vi "Search_Replace_File.vi"(2 "Replace_String":string="ADC Frequency Hz\t20000", 3 "Search_String":string="ADC Frequency Hz\t1000", 4 "Path":path) -> (0 "error out":errorcluster, 1 "Number Found":i32)   [LabVIEW 2010]
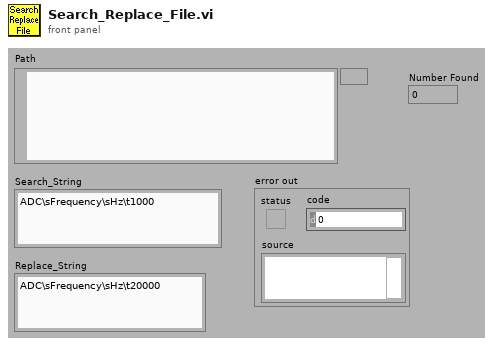
[diagram p1: front panel]
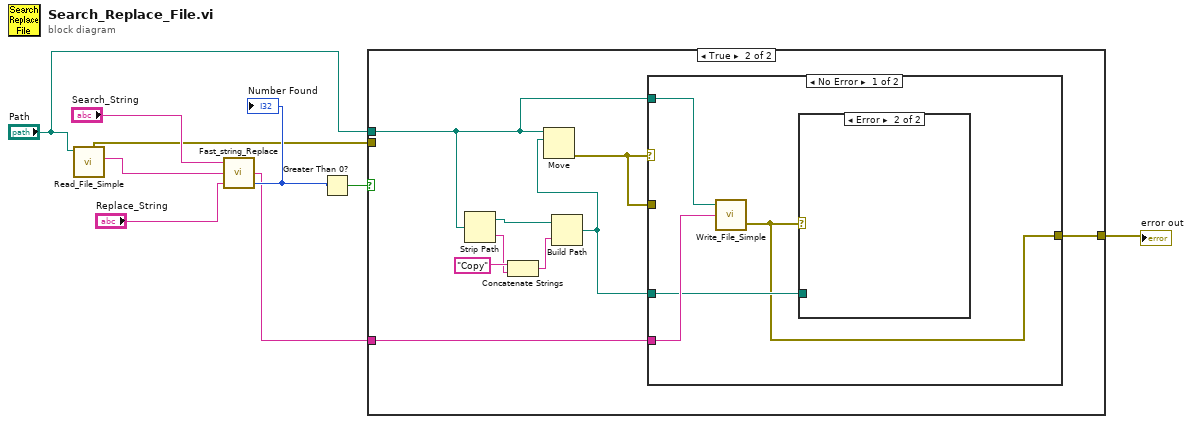
[diagram p0: block diagram]
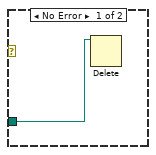
[diagram p3: hidden frame]
diagram:
  n1 = call "Read_File_Simple.vi"("Filename"="Path") -> ("error out"=w1:errorcluster, "string"=w9:string)  [unwired: 4 in, 4 out]
  n2 = call "Fast_string_Replace.vi"("Replace match with:"="Replace_String", "Input String"=w9, "regular expression"="Search_String") -> ("Number Found"=w6:i32, "Output String"=w3:string)  [unwired: 1 in]
  "Number Found" <- w6
  n3 = Greater Than 0?(x=w6) -> (x > 0?=w5:bool)
  n4 = case shown="True" w5 {
    tunnel: "Path" -> [_ w15]
    tunnel: w3 -> [_ w14]
    tunnel: [w10 w12] -> w2
    tunnel: w1 -> [w10 _]
    frame False {
    }
    frame True {
      n5 = Strip Path(path=w15) -> (stripped path=w16:path, name=w18:string)
      n6 = Concatenate Strings("Copy" ("name or relative path"), w18) -> (w17:string)
      n7 = Build Path(base path=w16, name or relative path=w17) -> (appended path=w13:path)
      n8 = Move(source path=w15, 10:w13) -> (error out=w11:errorcluster)  [unwired: 3 in, 2 out]
      n9 = case shown="No Error" w11 {
        tunnel: w15 -> [w23 _]
        tunnel: w14 -> [w22 _]
        tunnel: w13 -> [w21 _]
        tunnel: [w20 w25] -> w12
        tunnel: w11 -> [_ w25]
        frame No Error {
          n10 = call "Write_File_Simple.vi"("character string"=w22, "file path"=w23) -> ("error out"=w20:errorcluster)  [unwired: 1 in, 1 out]
          n11 = case shown="Error" w20 {
            tunnel: w21 -> [w24 _]
            frame No Error {
              n12 = Delete(path (use dialog)=w24) -> ()  [unwired: 4 in, 3 out]
            }
            frame Error {
            }
          }
        }
        frame Error {
        }
      }
    }
  }
  "error out" <- w2
